vi "MessageName.vi"() -> (2 "MessageName":string)   [LabVIEW 2020, in "CmdAnalog.lvlib"]
uses:
  CmdAnalog.lvlib
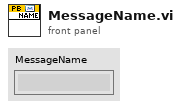
[diagram p1: front panel]
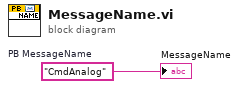
[diagram p0: block diagram]
diagram:
  w1 = "CmdAnalog"  # PB MessageName
  "MessageName" <- w1
